vi "set channel.vi"(8 "error in (no error)":errorcluster, 9 "Channel Data Reference":dbl, 10 "HW Chn":T2, 11 "Refnum in":T1) -> (0 "error out":errorcluster, 1 "coerced resistance (ohms)":dbl)   [LabVIEW 2017, in "NI 272x Resistive Simulation Custom Device Engine.lvlib"]
uses:
  NI 272x Resistive Simulation Custom Device Engine.lvlib
  Controls/Compiled HW Channel.ctl
  Controls/Channel Mode.ctl
  <instrlib>/ni272xReferenceVIs/ni272xReferenceVIs.llb/ni272x Callendar-Van Dusen RTD Parameters.ctl
  <instrlib>/ni272xReferenceVIs/ni272xReferenceVIs.llb/ni272x Reference.ctl
  <instrlib>/ni272xReferenceVIs/ni272xReferenceVIs.llb/ni272x Write Temperature 1Chan 1Samp.vi
  <instrlib>/ni272xReferenceVIs/ni272xReferenceVIs.llb/ni272x Write Resistance 1Chan 1Samp.vi
  NI 272x Resistive Simulation Custom Device Shared.lvlib
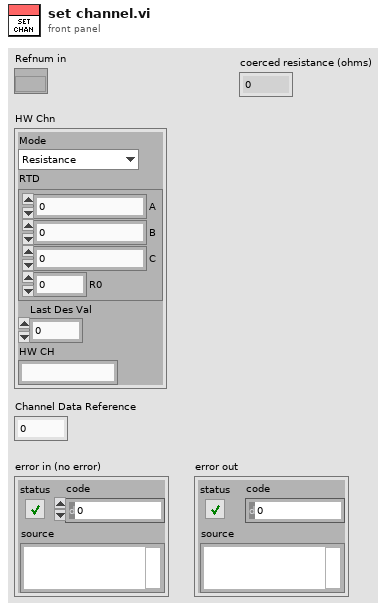
[diagram p1: front panel]
types:
  T1 = typedef "ni272x Reference.ctl" = refnum<k20>
  T2 = typedef "NI 272x Resistive Simulation Custom Device Shared.lvlib/Compiled HW Channel.ctl" = cluster{"Mode":T3, "RTD":T4, "Last Des Val":dbl, "HW CH":string}
  T3 = typedef "NI 272x Resistive Simulation Custom Device Shared.lvlib/Channel Mode.ctl" = enum16{"Resistance", "RTD Temperature"}
  T4 = typedef "ni272x Callendar-Van Dusen RTD Parameters.ctl" = cluster{"A":dbl, "B":dbl, "C":dbl, "R0":dbl}
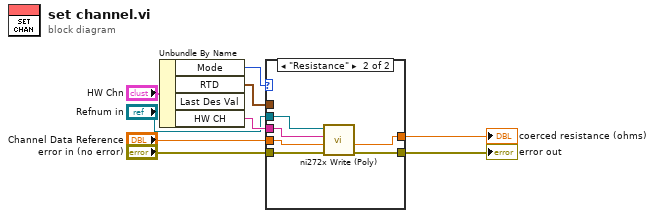
[diagram p0: block diagram]
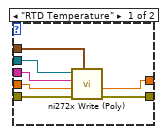
[diagram p2: hidden frame]
diagram:
  n1 = Unbundle By Name("HW Chn") -> ("Mode"=w4:T3, "RTD"=w7:T4, "HW CH"=w5:string)  [unwired: 1 out]
  n2 = case shown="\"Resistance\"" w4 {
    tunnel: "Refnum in" -> [w16 w22]
    tunnel: w5 -> [w15 w21]
    tunnel: "Channel Data Reference" -> [w14 w20]
    tunnel: w7 -> [w13 _]
    tunnel: [w11 w18] -> w9
    tunnel: "error in (no error)" -> [w12 w19]
    tunnel: [w10 w17] -> w1
    frame "RTD Temperature" {
      n3 = call-poly <instrlib>:"ni272x Write (Poly).vi"("Callendar-Van Dusen RTD parameters"=w13, "error in (no error)"=w12, "requested temperature (degrees Celsius)"=w14, "resistor channel"=w15, "instrument handle"=w16) -> ("error out"=w11:errorcluster, "coerced temperature (degrees Celsius)"=w10:dbl)  [unwired: 4 in, 1 out]
    }
    frame "Resistance" {
      n4 = call-poly <instrlib>:"ni272x Write (Poly).vi"("error in (no error)"=w19, "requested resistance (ohms)"=w20, "resistor channel"=w21, "instrument handle"=w22) -> ("error out"=w18:errorcluster, "coerced resistance (ohms)"=w17:dbl)  [unwired: 5 in, 1 out]
    }
  }
  "error out" <- w9
  "coerced resistance (ohms)" <- w1
